vi "Do.vi"(8 "error in":errorcluster, 10 "Actor in":refnum<class "Actor.lvclass">, 11 "Toggle Speaker Cycle MSG":refnum<class "Toggle Speaker Cycle MSG.lvclass">) -> (0 "error out":errorcluster, 2 "Actor out":refnum<class "Actor.lvclass">)   [LabVIEW 2014, in "Controller.lvlib" / "Toggle Speaker Cycle MSG.lvclass"]
doc: "(<B>Filename</B>: Actor Framework.lvlib:Message.lvclass:Do.vi)\n\nDefines what a message does when it is received by an actor. Generally, a message instructs an actor to invoke one of its methods. By default, this method does nothing. A child class must override it to define behavior. Create a child class by using the Actor Framework Message Maker dialog box."
uses:
  Toggle Speaker Cycle MSG.lvclass
  <vilib>/ActorFramework/Actor/Actor.lvclass
  Toggle Speaker Cycle MSG.lvclass/Toggle Speaker Cycle MSG.ctl
  Controller.lvclass
  SuperActor/Ex Nested.lvclass/Ex Nested.ctl
  Controls/Enqueuer Enum.ctl
  Instr Actor/Messages/Speaker Cycle MSG/Spk Cycle MSG.lvclass
  Instr Actor/Messages/Speaker Cycle MSG/Spk Cycle MSG.lvclass/Spk Cycle MSG.ctl
  Instr Actor/Messages/Speaker Cycle MSG/Write Cycle_.vi
  SuperActor/Read Log Session.vi
  <userlib>/_Session Fwk/Session - Root.lvclass
  reusable/Session APIs/Session Log/System Log.lvclass
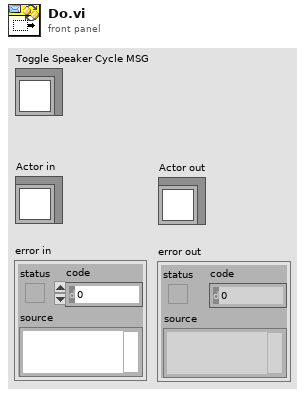
[diagram p1: front panel]
types:
  T1 = typedef "Enqueuer Enum.ctl" = enum8{"PAS", "CRDS", "File"}
  T2 = typedef "Session - Root.lvclass/Session Handle.ctl" = refnum<data-value>
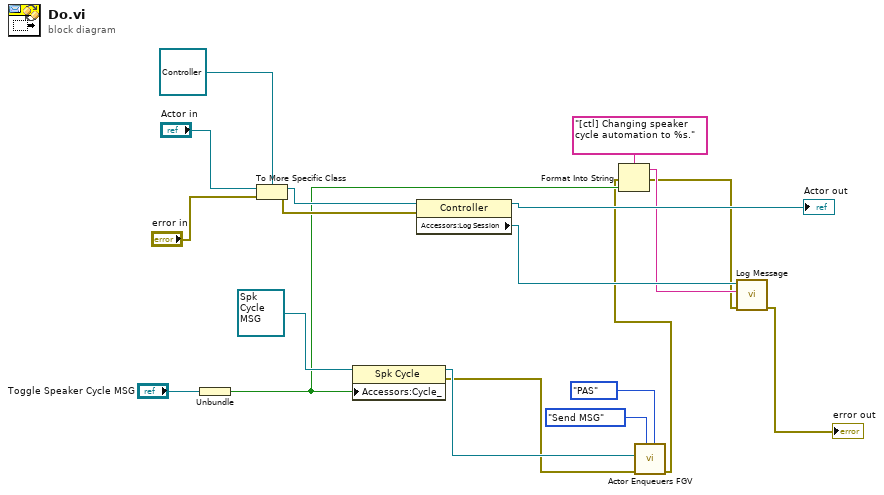
[diagram p0: block diagram]
diagram:
  n1 = Unbundle("Toggle Speaker Cycle MSG") -> (w4:bool)
  n2 = To More Specific Class(target class=refnum<class "Controller.lvclass"> refnum ("Controller:Controller"), reference="Actor in", error in="error in") -> (specific class reference=w10:refnum<class "Controller.lvclass">, error out=w9:errorcluster)
  n3 = property class="Spk Cycle"(reference=refnum<class "Spk Cycle MSG.lvclass"> refnum ("ePAS Library.lvlib:Spk Cycle"), "Accessors:Cycle_"=w4) -> (reference out=w12:refnum<class "Spk Cycle MSG.lvclass">, error out=w11:errorcluster)  [unwired: 1 in]
  n4 = property class="Controller"(reference=w10, error in=w9) -> (reference out=→"Actor out":refnum<class "Controller.lvclass">, "Accessors:Log Session"=w8:T2)  [unwired: 1 out]
  n5 = call "Actor Enqueuers FGV.vi"("Enqueuer"=Enqueuer_Enum."PAS", "State"=enum16{"Store", "Send MSG"}."Send MSG", "error in"=w11, "MSG"=w12) -> ("error out"=w2:errorcluster)  [unwired: 7 in]
  n6 = Format Into String(format string="[ctl] Changing speaker cycle automation to %s.", error in=w2, w4) -> (resulting string=w3:string, error out=w1:errorcluster)  [unwired: 1 in]
  n7 = call "Log Message.vi"("error in"=w1, "MSG In"=w3, "session in"=w8) -> ("error out"=→"error out":errorcluster)  [unwired: 7 in, 1 out]
